vi "closeDelta.vi"(8 "error in (no error)":errorcluster, 11 "VISA Refnum in":refnum<visa-resource-name>) -> (0 "error out":errorcluster)   [LabVIEW 2012]
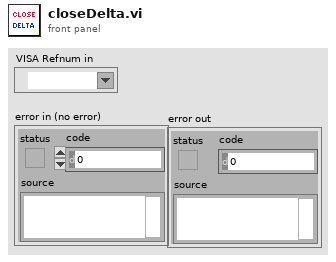
[diagram p1: front panel]
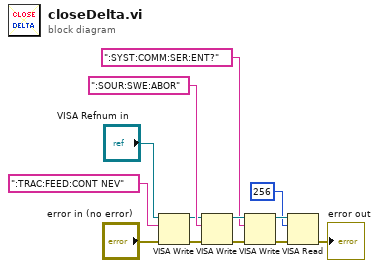
[diagram p0: block diagram]
diagram:
  n1 = VISA Write(VISA resource name="VISA Refnum in", write buffer=":TRAC:FEED:CONT NEV" ("format string"), error in (no error)="error in (no error)") -> (VISA resource name out=w3:refnum<visa-resource-name>, error out=w5:errorcluster)  [unwired: 1 out]
  n2 = VISA Write(VISA resource name=w3, write buffer=":SOUR:SWE:ABOR" ("format string"), error in (no error)=w5) -> (VISA resource name out=w10:refnum<visa-resource-name>, error out=w11:errorcluster)  [unwired: 1 out]
  n3 = VISA Write(VISA resource name=w10, write buffer=":SYST:COMM:SER:ENT?" ("format string"), error in (no error)=w11) -> (VISA resource name out=w12:refnum<visa-resource-name>, error out=w13:errorcluster)  [unwired: 1 out]
  n4 = VISA Read(VISA resource name=w12, byte count=u32 256 ("Max Num Bytes To Read (256)"), error in (no error)=w13) -> (error out=→"error out":errorcluster)  [unwired: 3 out]
